vi "Single Sweep.vi"(8 "error in (no error)":errorcluster, 11 "VISA resource name":refnum<visa-resource-name>) -> (0 "error out":errorcluster, 3 "VISA resource name out":refnum<visa-resource-name>)   [LabVIEW 2012, in "Agilent PSG MXG Series.lvlib"]
doc: "Aborts the current sweep, and then either arms or arms and starts a single list, step, or ramp sweep (Option 007), depending on the trigger type.\n\n<B>Notes:</B>\n(1) This VI is valid only in E8247C, E8257C, E8267C, E8257D, E8267D, N5161A, N5162A, N5181A, N5182A, N5183A, N5171B, N5172B, N5181B, N5182B.\n\n(2) Arms a single sweep when the trigger source selection is Bus, External, or Key. Arms or starts a single sweep when the trigger source selection is Immediate."
uses:
  <instrlib>/Agilent PSG MXG Series/Agilent PSG MXG Series.lvlib
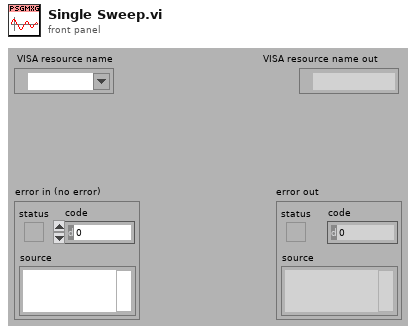
[diagram p1: front panel]
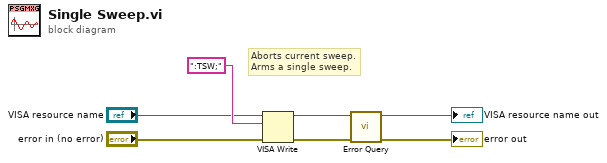
[diagram p0: block diagram]
diagram:
  # "Aborts current sweep.\nArms a single sweep."
  n1 = VISA Write(VISA resource name="VISA resource name", write buffer=":TSW;", error in (no error)="error in (no error)") -> (VISA resource name out=w6:refnum<visa-resource-name>, error out=w5:errorcluster)  [unwired: 1 out]
  n2 = call <instrlib>:"Error Query.vi"("error in (no error)"=w5, "VISA resource name"=w6) -> ("error out"=→"error out":errorcluster, "VISA resource name out"=→"VISA resource name out":refnum<visa-resource-name>)  [unwired: 8 out]
